vi "photometry_15.vi"() -> ()   [LabVIEW 2013]
doc: "This example demonstrates how to continuously acquire buffered voltage measurements using a DAQmx device.\n\nFor instructions on how to connect your signals to the DAQ device, refer to your device documentation."
uses:
  <vilib>/Utility/error.llb/DialogType.ctl
  <vilib>/Platform/TimedLoop/XDataNode/timing_clust.ctl
  <vilib>/Platform/TimedLoop/XDataNode/nitl_modes.ctl
  <vilib>/Platform/TimedLoop/XDataNode/wakeup.ctl
  <vilib>/DAQmx/write.llb/DAQmx Write (Analog 1D Wfm NChan NSamp).vi
  <vilib>/DAQmx/read.llb/DAQmx Read (Analog 1D Wfm NChan NSamp).vi
  <vilib>/DAQmx/create/channels.llb/DAQmx Create Channel (AI-Voltage-Basic).vi
  <vilib>/DAQmx/configure/timing.llb/DAQmx Timing (Sample Clock).vi
  <vilib>/DAQmx/miscellaneous.llb/DAQmx Fill In Error Info.vi
  <vilib>/DAQmx/create/channels.llb/DAQmx Create Channel (AO-Voltage-Basic).vi
  <vilib>/platform/TimedLoop/XDataNode/XDataNode.xnode
  <resource>/objmgr/daqmx.rc
  <vilib>/Platform/TimedLoop/XDataNode/XDNodeRunTimeDep.lvlib
  <vilib>/measure/NI_MABase.lvlib
panel:
  out "Offsets Local Variable":dbl[](array[numeric]) caption="Offset" step=0.1
  in  "LED Driver\nmA max":dbl[](array[numeric])=[0.0, 0.0] caption="LED Driver max (mA)" step=0.1
  in  "Offset":dbl[](array[numeric])=[0.0, 0.0] step=0.1
  out "current  output":dbl[](array[numeric])
  out "raw signal [min max]":string
  out "UV graph avg":dbl
  out "blue graph avg":dbl
  out "Waveform Chart 2":dynamicdata(graph)
  out "Waveform Chart":dynamicdata(graph)
  out "ampl local variable":dbl[](array[numeric]) caption="Amplitude (V)"
  in  "Phase (Deg)":dbl[](array[numeric])=[0.0, 0.0]
  in  "Waveform Type":T1(array[ring])=[enum."Sine Wave", enum."Sine Wave"]
  in  "Sample Clock Rate":dbl=10000.0 caption="AO Sampl Rate" format="%.2f"
  in  "Desired Frequency":dbl[](array[numeric])=[211.0, 500.0] caption="Freq (Hz)"
  in  "Samples per Buffer":dbl=10000.0 caption="AO Sampl/\nBuffer"
  in  "Amplitude":dbl[](array[numeric])=[0.0, 0.0] caption="Amplitude (V)" step=0.1
  out "Output Data":waveform(dbl)[](graph)
  in  "Physical Channels":tag="Dev2/ao0:1"
  in  "Minimum Value":dbl caption="Max V" format="%0.2f"
  in  "Maximum Value":dbl=5.0 caption="Min V" format="%0.2f"
  out "?":bool
  in  "Input sampl rate":dbl=10000.0
  in  "session name (optional;\nno special chars)":string
  in  "output folder":path=path "D:/photometry/data"
  in  "?":bool
  out "Time":string caption="Elapsed Time Text"
  in  "Input nr samples":i32=10000
  in  "Terminal Configuration":i32(ring)=10083 items=["default"=-1, "RSE"=10083, "NRSE"=10078, "Differential"=10106, "Pseudodifferential"=12529]
  in  "Max Voltage":dbl=5.0
  in  "Min Voltage":dbl=-5.0
  in  "?":string="Dev2/ai0:2,Dev2/ai5"
  out "Actual Sample Rate":dbl=1000.0 format="%0.2f"
  # "Inputs to demodulator"
  # "Channel Configuration"
  # "Demodulated Signal"
  # "Input Channels"
  # "LED parameters"
  # "Blue"
  # "UV"
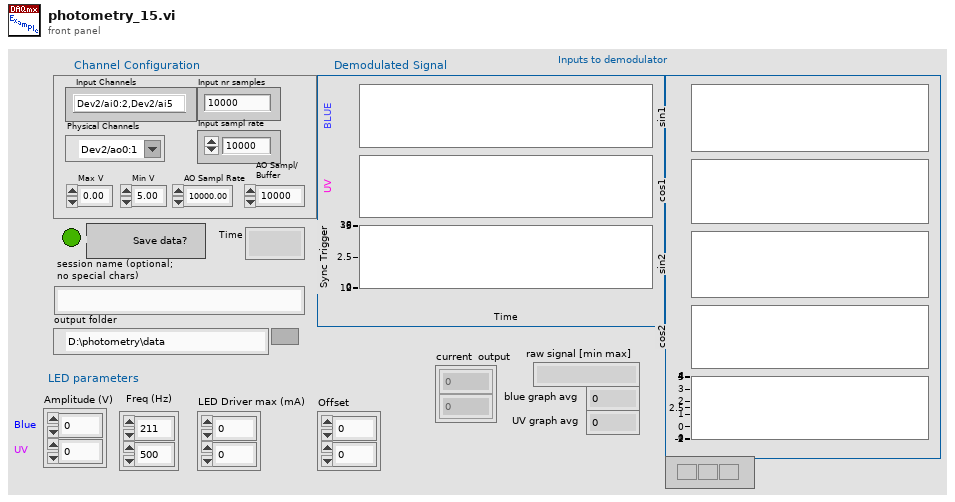
[diagram p1: front panel]
types:
  T1 = enum16{"Sine Wave", "Triangle Wave", "Square Wave", "Sawtooth Wave"}[]
  T2 = typedef "DialogType.ctl" = u16
  T3 = typedef "XDNodeRunTimeDep.lvlib/timing_clust.ctl" = cluster{"Expected End [f-1]":u64, "Actual End [f-1]":u64, "Finished Late? [f-1]":bool, "Expected End [i-1]":u64, "Actual End [i-1]":u64, "Finished Late? [i-1]":bool, "Expected Start [i]":u64, "Actual Start [i]":u64, "Expected Start [f]":u64, "Actual Start [f]":u64, "Source Name":string, "Structure Name":string, "Period":i64, "Deadline":i64, "Offset":i64, "Start":i64, "Priority":i32, "Timeout":i32, "Mode":T4, "Wakeup Reason":T5, "Error":errorcluster, "Source Type":string, "Secondary Source Type":string, "Global End Time":u64, "Global Start Time":u64, "Frame Duration":u64, "Iteration Duration":u64, "Assigned CPU":i32, "I/O Scan Engine Mode":u32}
  T4 = typedef "XDNodeRunTimeDep.lvlib/nitl_modes.ctl" = enum32{"No Change", "Process missed periods, maintain original phase", "Discard missed periods, maintain original phase", "Process missed periods, ignore original phase", "Discard missed periods, ignore original phase"}
  T5 = typedef "XDNodeRunTimeDep.lvlib/wakeup.ctl" = enum32{"Normal", "Aborted", "Asynchronous wakeup", "Timing source error", "Timed loop error", "Timeout"}
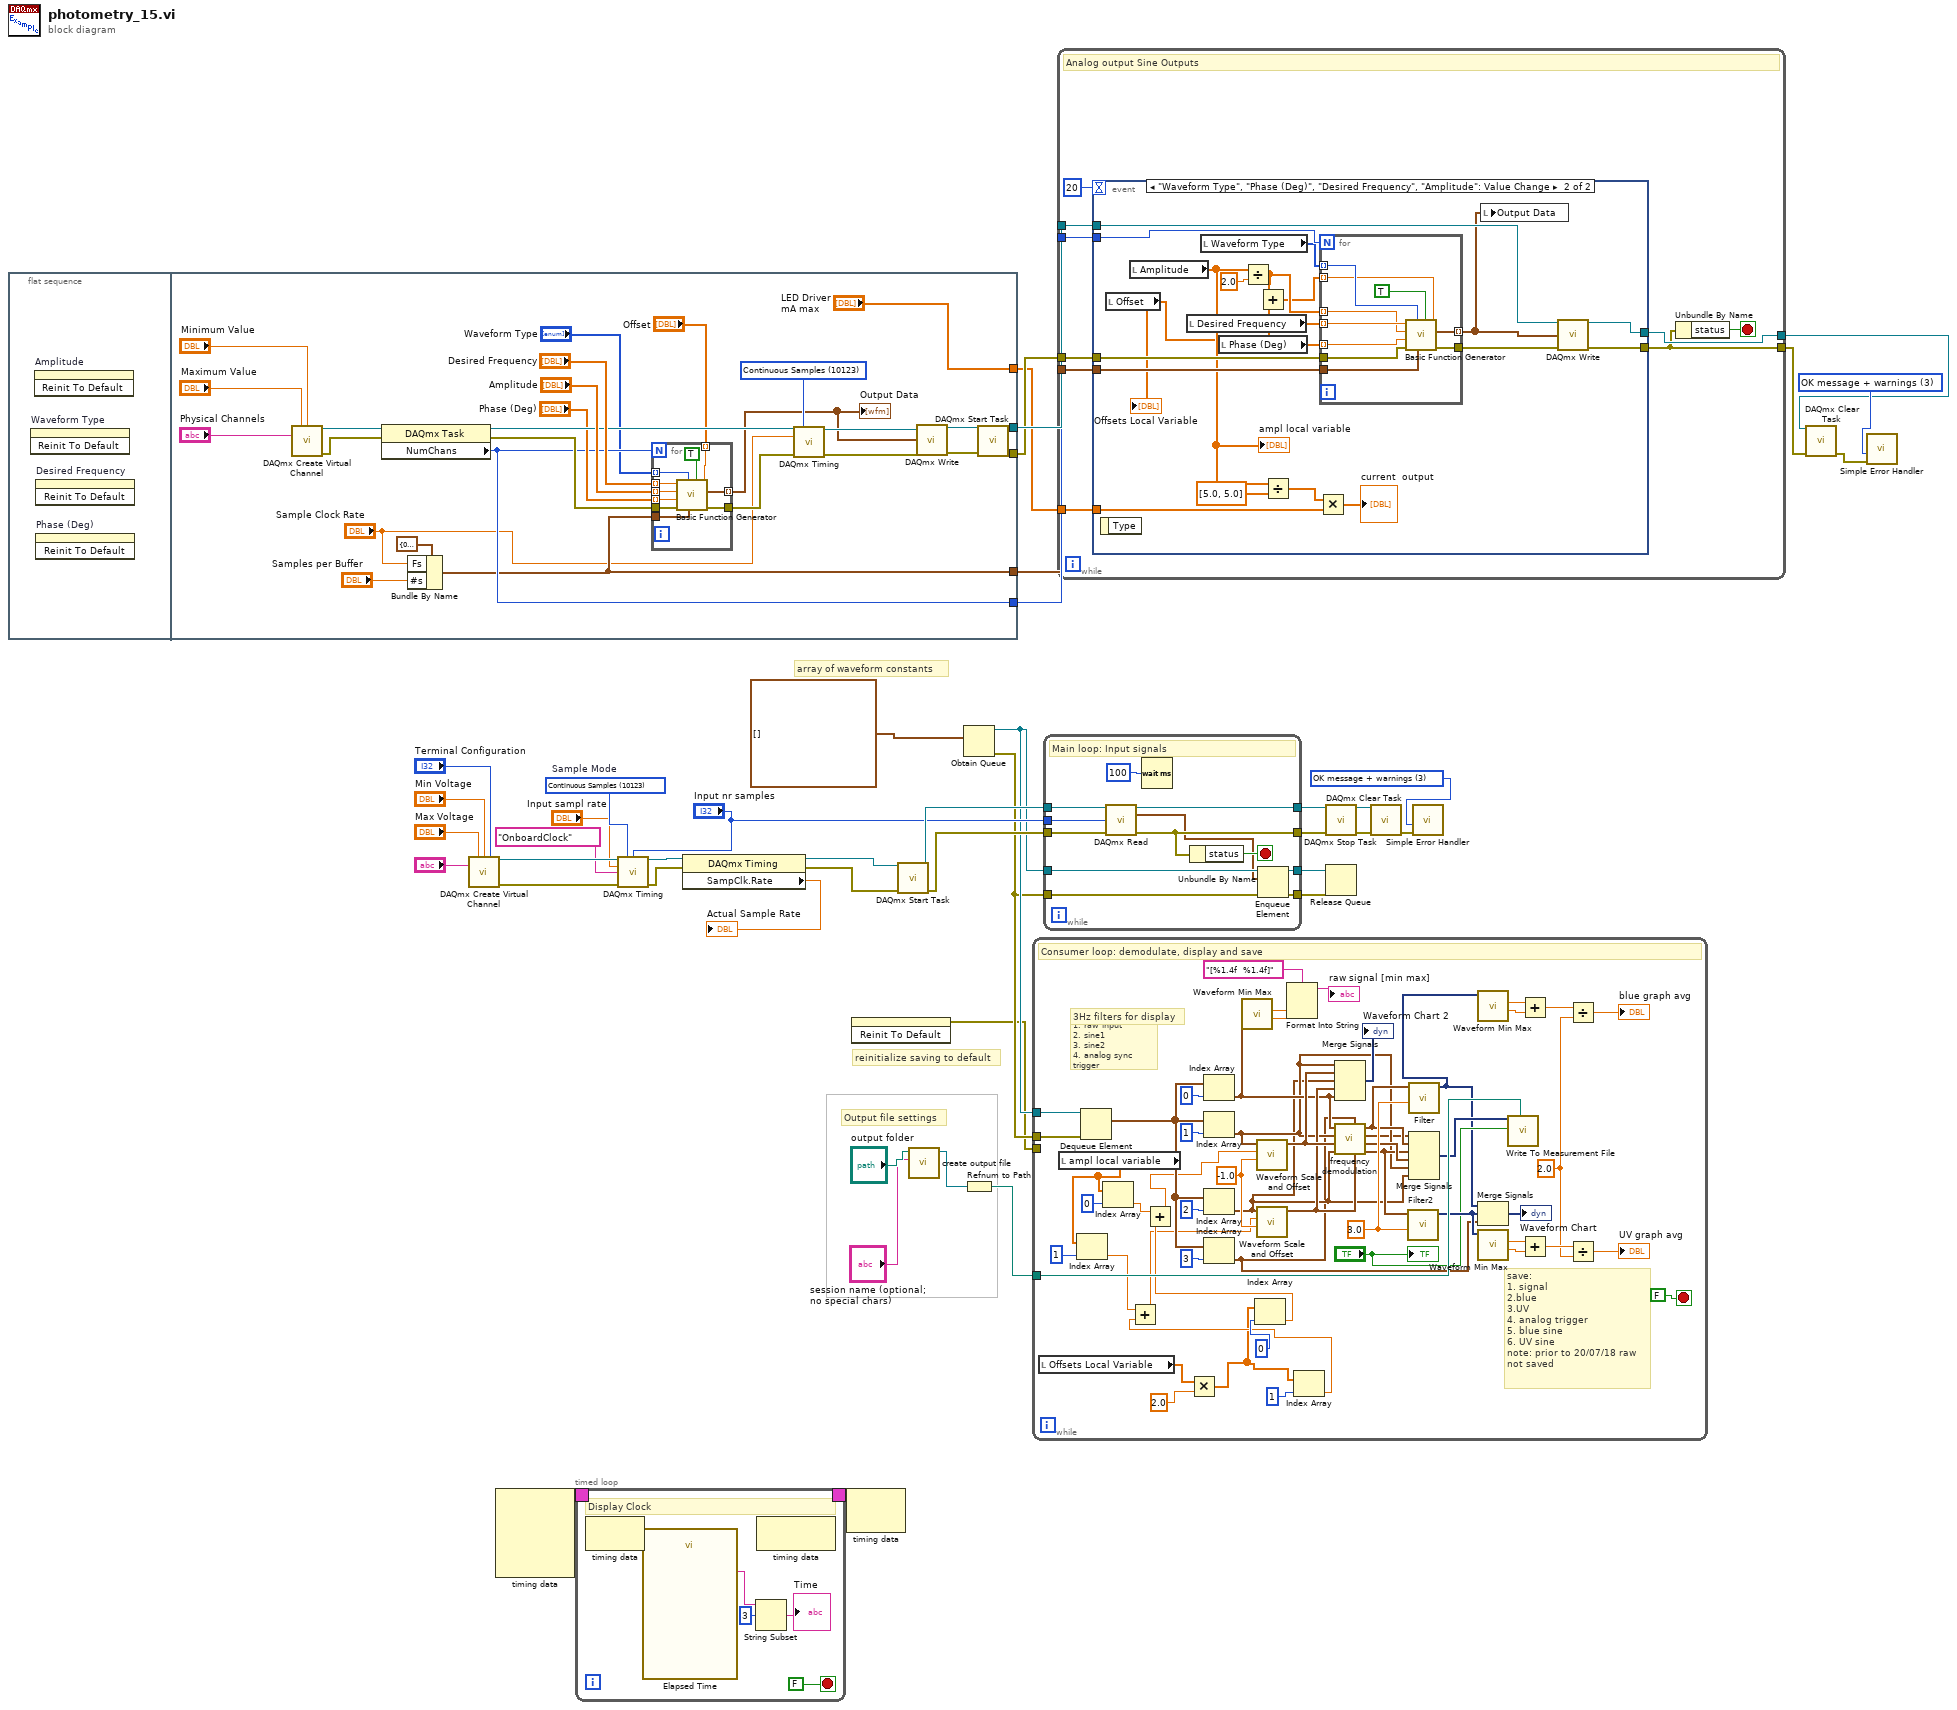
[diagram p0: block diagram]
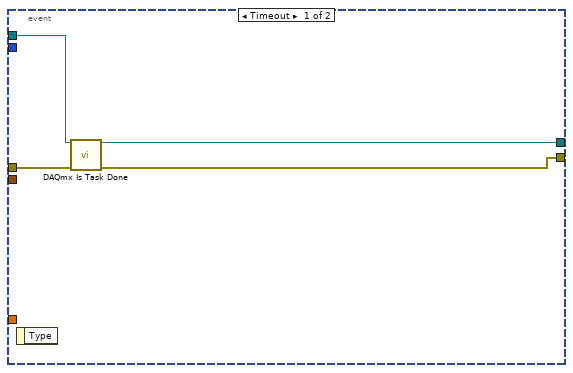
[diagram p2: hidden frame]
diagram:
  w7 = T2 3 items=["no dialog", "OK message", "continue or stop message", "OK message + warnings", "continue/stop + warnings"] ("type of dialog (OK msg:1)")
  w24 = T2 3 items=["no dialog", "OK message", "continue or stop message", "OK message + warnings", "continue/stop + warnings"] ("type of dialog (OK msg:1)")
  w42 = 10123 items=["Finite Samples"=10178, "Continuous Samples"=10123, "Hardware Timed Single Point"=12522]  # Sample Mode
  # "array of waveform constants"
  # "Output file settings"
  # "reinitialize saving to default"
  n1 = flat-sequence {
    tunnel: [w71] -> w9
    tunnel: [w65] -> w8
    tunnel: [w50] -> w6
    tunnel: [w48] -> w3
    tunnel: ["LED Driver\nmA max"] -> w1
    frame #0 {
      n2 = invoke on="Waveform Type" class="Arr (strict)" method="Reinit To Default"() -> ()  [unwired: 3 in, 3 out]
      n3 = invoke on="Amplitude" class="Arr (strict)" method="Reinit To Default"() -> ()  [unwired: 3 in, 3 out]
      n4 = invoke on="Desired Frequency" class="Arr (strict)" method="Reinit To Default"() -> ()  [unwired: 3 in, 3 out]
      n5 = invoke on="Phase (Deg)" class="Arr (strict)" method="Reinit To Default"() -> ()  [unwired: 3 in, 3 out]
    }
    frame #1 {
      w70 = 10123 items=["Finite Samples"=10178, "Continuous Samples"=10123] ("sample mode")
      n6 = call-poly <vilib>:"DAQmx Create Virtual Channel.vi"("maximum value"="Maximum Value", "minimum value"="Minimum Value", "physical channels"="Physical Channels") -> ("task out"=w56:refnum<k21>, "error out"=w52:errorcluster)  [unwired: 11 in]
      n7 = property class="DAQmx Task"(reference=w56, error in=w52) -> (reference out=w55:refnum<k21>, error out=w54:errorcluster, "NumChans"=w50:u32)
      n8 = Bundle By Name(cluster=cluster{"Fs":dbl, "#s":dbl} {"Fs"=0.0, "#s"=0.0} ("sampling info"), "Fs"="Sample Clock Rate", "#s"="Samples per Buffer") -> (w48:cluster{"Fs":dbl, "#s":dbl})
      n9 = for {
        N: w50 -> [_]
        tunnel: "Amplitude" -> [w81] mode=indexing
        tunnel: "Desired Frequency" -> [w80] mode=indexing
        tunnel: [w79] -> w57
        tunnel: w54 -> [w78]
        tunnel: [w77] -> w53 mode=indexing
        tunnel: "Phase (Deg)" -> [w76] mode=indexing
        tunnel: w48 -> [w74]
        tunnel: "Waveform Type" -> [w73] mode=indexing
        tunnel: "Offset" -> [w72] mode=indexing
        n10 = call <vilib>:"Basic Function Generator.vi"("offset"=w72, "reset signal"=TRUE, "sampling info"=w74, "signal type"=w73, "error in (no error)"=w78, "phase"=w76, "amplitude"=w81, "frequency"=w80) -> ("error out"=w79:errorcluster, "signal out"=w77:waveform(dbl))  [unwired: 1 in, 1 out]
      }
      "Output Data" <- w53
      n11 = call-poly <vilib>:"DAQmx Timing.vi"("task/channels in"=w55, "sample mode"=w70, "rate"="Sample Clock Rate", "error in"=w57) -> ("task out"=w64:refnum<k21>, "error out"=w62:errorcluster)  [unwired: 10 in]
      n12 = call-poly <vilib>:"DAQmx Write.vi"("task/channels in"=w64, "data"=w53, "error in"=w62) -> ("task out"=w67:refnum<k21>, "error out"=w66:errorcluster)  [unwired: 10 in, 1 out]
      n13 = call <vilib>:"DAQmx Start Task.vi"("task/channels in"=w67, "error in"=w66) -> ("task out"=w71:refnum<k21>, "error out"=w65:errorcluster)  [unwired: 12 in]
    }
  }
  n14 = call-poly <vilib>:"DAQmx Create Virtual Channel.vi"("maximum value"="Max Voltage", "minimum value"="Min Voltage", "input terminal configuration"="Terminal Configuration", "physical channels"="?") -> ("task out"=w40:refnum<k21>, "error out"=w41:errorcluster)  [unwired: 10 in]
  n15 = node-c288() -> (w23:T3)  [unwired: 4 in]
  n16 = timed-loop {
    timing: w23 -> [_]
    timing-out: [_] -> w22
    stop <- FALSE stop-if-true
    # "Display Clock"
    n17 = node-c288() -> ()  [unwired: 1 in, 1 out]
    n18 = call "Elapsed Time"() -> ("Elapsed Time Text"=w83:string)  [unwired: 12 in, 7 out]
    n19 = String Subset(string=w83, offset (0)=3) -> (substring=→"Time":string)  [unwired: 1 in]
    n20 = node-c288() -> ()  [unwired: 1 in, 1 out]
  }
  n21 = call-poly <vilib>:"DAQmx Timing.vi"("task/channels in"=w40, "sample mode"=w42, "samples per channel"="Input nr samples", "rate"="Input sampl rate", "source"=tag "OnboardClock" ("Sample Clock Source"), "error in"=w41) -> ("task out"=w44:refnum<k21>, "error out"=w43:errorcluster)  [unwired: 8 in]
  n22 = property class="DAQmx Timing"(reference=w44, error in=w43) -> (reference out=w12:refnum<k21>, error out=w11:errorcluster, "SampClk.Rate"=→"Actual Sample Rate":dbl)
  n23 = node-c288(w22) -> ()  [unwired: 1 out]
  n24 = invoke class="Bool (strict)" method="Reinit To Default"() -> (error out=w17:errorcluster)  [unwired: 3 in, 2 out]
  n25 = call <vilib>:"DAQmx Start Task.vi"("task/channels in"=w12, "error in"=w11) -> ("task out"=w39:refnum<k21>, "error out"=w38:errorcluster)  [unwired: 12 in]
  n26 = call "create output file.vi"("session name\n(optional; no special characters)"="session name (optional;\nno special chars)", "input path"="output folder") -> ("refnum out"=w14:refnum<file>)  [unwired: 9 in]
  n27 = Obtain Queue(element data type=waveform(dbl)[] [] ("waveform array")) -> (queue out=w19:refnum<queue>, error out=w18:errorcluster)  [unwired: 4 in, 1 out]
  n28 = Refnum to Path(1:w14) -> (0:w13:path)
  n29 = while {
    tunnel: w19 -> [w141]
    tunnel: w18 -> [w140]
    tunnel: w17 -> [_]
    tunnel: w13 -> [w139]
    stop <- FALSE stop-if-true
    w116 = -1.0 ("scale")
    w135 = 3.0 ("Lower Cut-Off")
    w122 = 2.0 ("y")
    # "save:\n1. signal\n2.blue\n3.UV\n4. analog trigger\n5. blue sine\n6. UV sine\nnote: prior to 20/07/18 raw not saved"
    # "input signals are:\n1. raw input\n2. sine1\n3. sine2\n4. analog sync trigger"
    # "3Hz filters for display"
    # "Consumer loop: demodulate, display and save"
    n30 = local read "Offsets Local Variable"() -> (w89:dbl[])
    n31 = local read "ampl local variable"() -> (w103:dbl[])
    n32 = Index Array(array=w103, index=1) -> (element=w93:dbl)
    n33 = Dequeue Element(queue=w141, error in (no error)=w140) -> (element=w118:waveform(dbl)[])  [unwired: 1 in, 3 out]
    n34 = Index Array(array=w103, index=0) -> (element=w96:dbl)
    n35 = Multiply(x=w89, y=2.0) -> (x*y=w90:dbl[])
    n36 = Index Array(array=w118, index=0) -> (element=w112:waveform(dbl))
    n37 = Index Array(array=w118, index=1) -> (element=w107:waveform(dbl))
    n38 = Index Array(array=w118, index=2) -> (element=w106:waveform(dbl))
    n39 = Index Array(array=w118, index=3) -> (element=w100:waveform(dbl))
    n40 = call <vilib>:"Waveform Min Max.vi"("waveform in"=w112) -> ("Y min"=w125:dbl, "Y max"=w126:dbl)  [unwired: 5 in, 4 out]
    n41 = Index Array(array=w90, index=0) -> (element=w94:dbl)
    n42 = Add(x=w96, y=w94) -> (x+y=w95:dbl)
    n43 = call <vilib>:"Waveform Scale and Offset.vi"("scale"=w116, "offset"=w95, "waveform in"=w107) -> ("waveform out"=w115:waveform(dbl))  [unwired: 7 in, 1 out]
    n44 = Format Into String(format string="[%1.4f  %1.4f]", w126, w125) -> (resulting string=→"raw signal [min max]":string)  [unwired: 2 in, 1 out]
    n45 = Index Array(array=w90, index=1) -> (element=w92:dbl)
    n46 = Add(x=w93, y=w92) -> (x+y=w91:dbl)
    n47 = call <vilib>:"Waveform Scale and Offset.vi"("scale"=w116, "offset"=w91, "waveform in"=w106) -> ("waveform out"=w114:waveform(dbl))  [unwired: 7 in, 1 out]
    n48 = Merge Signals(w107, w115, w106, w114, w112) -> (→"Waveform Chart 2":dynamicdata)
    n49 = call "frequency demodulation.vi"("signal"=w112, "210Hz sine"=w107, "210Hz cosine"=w115, "500Hz sine"=w106, "analog trigger in"=w100, "500 Hz cosine"=w114) -> ("blue"=w110:waveform(dbl), "raw signal out"=w99:waveform(dbl), "analog trig out"=w109:waveform(dbl), "uv"=w108:waveform(dbl))
    n50 = call "Filter2"("Lower Cut-Off"=w135, "Signal"=w108) -> ("Filtered Signal"=w113:dynamicdata)  [unwired: 8 in, 1 out]
    n51 = call "Filter"("Lower Cut-Off"=w135, "Signal"=w110) -> ("Filtered Signal"=w101:dynamicdata)  [unwired: 8 in, 1 out]
    n52 = Merge Signals(w99, w110, w108, w109, w107, w106) -> (w105:dynamicdata)
    n53 = call <vilib>:"Waveform Min Max.vi"("waveform in"=w101) -> ("Y min"=w127:dbl, "Y max"=w128:dbl)  [unwired: 5 in, 4 out]
    n54 = Merge Signals(w101, w113, w100) -> (→"Waveform Chart":dynamicdata)
    n55 = call <vilib>:"Waveform Min Max.vi"("waveform in"=w113) -> ("Y min"=w129:dbl, "Y max"=w130:dbl)  [unwired: 5 in, 4 out]
    n56 = call "Write To Measurement File"("Signals"=w105, "Enable"="?", "Filename"=w139) -> ()  [unwired: 14 in, 3 out]
    n57 = Add(x=w128, y=w127) -> (x+y=w134:dbl)
    n58 = Add(x=w130, y=w129) -> (x+y=w132:dbl)
    n59 = Divide(x=w134, y=w122) -> (x/y=→"blue graph avg":dbl)
    n60 = Divide(x=w132, y=w122) -> (x/y=→"UV graph avg":dbl)
    "?" <- "?"
  }
  n61 = while {
    tunnel: w39 -> [w153]
    tunnel: w38 -> [w152]
    tunnel: [w151] -> w28
    tunnel: [w150] -> w27
    tunnel: "Input nr samples" -> [w149]
    tunnel: w19 -> [w148]
    tunnel: w18 -> [w147]
    tunnel: [w146] -> w21
    tunnel: [w145] -> w20
    stop <- w144 stop-if-true
    # "Main loop: Input signals"
    n62 = call-poly <vilib>:"DAQmx Read.vi"("task/channels in"=w153, "number of samples per channel"=w149, "error in"=w152) -> ("task out"=w151:refnum<k21>, "data"=w142:waveform(dbl)[], "error out"=w150:errorcluster)  [unwired: 10 in]
    n63 = Wait (ms)(milliseconds to wait=u32 100) -> ()  [unwired: 1 out]
    n64 = Unbundle By Name(w150) -> ("status"=w144:bool)
    n65 = Enqueue Element(queue=w148, element=w142, error in (no error)=w147) -> (queue out=w146:refnum<queue>, error out=w145:errorcluster)  [unwired: 1 in, 1 out]
  }
  n66 = while {
    tunnel: w9 -> [w161]
    tunnel: w8 -> [w160]
    tunnel: w3 -> [w159]
    tunnel: w6 -> [w158]
    tunnel: [w157] -> w5
    tunnel: [w156] -> w4
    tunnel: w1 -> [w154]
    stop <- w155 stop-if-true
    # "Analog output Sine Outputs"
    n67 = event shown="[1] \"Waveform Type\", \"Phase (Deg)\", \"Desired Frequency\", \"Amplitude\": Value Change" {
      selector: _ -> [_ _]
      dyn-events: _ -> [_ _]
      timeout: 20 -> [_ _]
      tunnel: w161 -> [w166 w186]
      tunnel: w160 -> [w165 w185]
      tunnel: w159 -> [_ w177]
      tunnel: [w164 w181] -> w157
      tunnel: [w163 w180] -> w156
      tunnel: w158 -> [_ w178]
      tunnel: w154 -> [_ w172]
      event Timeout {
        n68 = event-data() -> ()  [unwired: 1 in, 1 out]
        n69 = call <vilib>:"DAQmx Is Task Done.vi"("task/channels in"=w166, "error in"=w165) -> ("task out"=w164:refnum<k21>, "error out"=w163:errorcluster)  [unwired: 11 in, 1 out]
      }
      event "Waveform Type", "Phase (Deg)", "Desired Frequency", "Amplitude": Value Change {
        n70 = event-data() -> ()  [unwired: 1 in, 1 out]
        n71 = local read "Offset"() -> (w168:dbl[])
        "Offsets Local Variable" <- w168
        n72 = local read "Amplitude"() -> (w174:dbl[])
        "ampl local variable" <- w174
        n73 = local read "Desired Frequency"() -> (w183:dbl[])
        n74 = local read "Waveform Type"() -> (w176:T1)
        n75 = local read "Phase (Deg)"() -> (w182:dbl[])
        n76 = Divide(x=w174, y=2.0) -> (x/y=w169:dbl[])
        n77 = Add(x=w169, y=w168) -> (x+y=w167:dbl[])
        n78 = Divide(x=w174, y=dbl[] [5.0, 5.0]) -> (x/y=w173:dbl[])
        n79 = Multiply(x=w173, y=w172) -> (x*y=→"current  output":dbl[])
        n80 = for {
          N: w178 -> [_]
          tunnel: [w196] -> w184
          tunnel: [w195] -> w179 mode=indexing
          tunnel: w185 -> [w194]
          tunnel: w183 -> [w193] mode=indexing
          tunnel: w169 -> [w192] mode=indexing
          tunnel: w182 -> [w191] mode=indexing
          tunnel: w177 -> [w189]
          tunnel: w176 -> [w188] mode=indexing
          tunnel: w167 -> [w187] mode=indexing
          n81 = call <vilib>:"Basic Function Generator.vi"("offset"=w187, "reset signal"=TRUE, "sampling info"=w189, "signal type"=w188, "error in (no error)"=w194, "phase"=w191, "amplitude"=w192, "frequency"=w193) -> ("error out"=w196:errorcluster, "signal out"=w195:waveform(dbl))  [unwired: 1 in, 1 out]
        }
        n82 = local write "Output Data"(w179) -> ()
        n83 = call-poly <vilib>:"DAQmx Write.vi"("task/channels in"=w186, "data"=w179, "error in"=w184) -> ("task out"=w181:refnum<k21>, "error out"=w180:errorcluster)  [unwired: 10 in, 1 out]
      }
    }
    n84 = Unbundle By Name(w156) -> ("status"=w155:bool)
  }
  n85 = call <vilib>:"DAQmx Stop Task.vi"("task/channels in"=w28, "error in"=w27) -> ("task out"=w25:refnum<k21>, "error out"=w26:errorcluster)  [unwired: 12 in]
  n86 = Release Queue(queue=w21, error in (no error)=w20) -> ()  [unwired: 1 in, 3 out]
  n87 = call <vilib>:"DAQmx Clear Task.vi"("task in"=w25, "error in"=w26) -> ("error out"=w37:errorcluster)  [unwired: 13 in]
  n88 = call <vilib>:"Simple Error Handler.vi"("type of dialog (OK msg:1)"=w24, "error in (no error)"=w37) -> ()  [unwired: 3 in, 5 out]
  n89 = call <vilib>:"DAQmx Clear Task.vi"("task in"=w5, "error in"=w4) -> ("error out"=w10:errorcluster)  [unwired: 13 in]
  n90 = call <vilib>:"Simple Error Handler.vi"("type of dialog (OK msg:1)"=w7, "error in (no error)"=w10) -> ()  [unwired: 3 in, 5 out]
